vi "Configure Generator State.vi"(8 "error in (no error)":errorcluster, 9 "State (Off)":bool, 10 "Instance (1)":i32=1 format="%.0g", 11 "VISA resource name":refnum<visa-resource-name>) -> (0 "error out":errorcluster, 3 "VISA resource name out":refnum<visa-resource-name>)   [LabVIEW 2020, in "Rohde&Schwarz CMXP GPRF.lvlib"]
doc: "Turns the generator on or off.\n\nAttribute:\nRSCMXPGPRF_ATTR_GENERATOR_STATE\n\nRemote-control command:\nSOURce:GPRF:GEN<i>:STATe"
uses:
  <instrlib>/Rohde&Schwarz CMXP GPRF/Rohde&Schwarz CMXP GPRF.lvlib
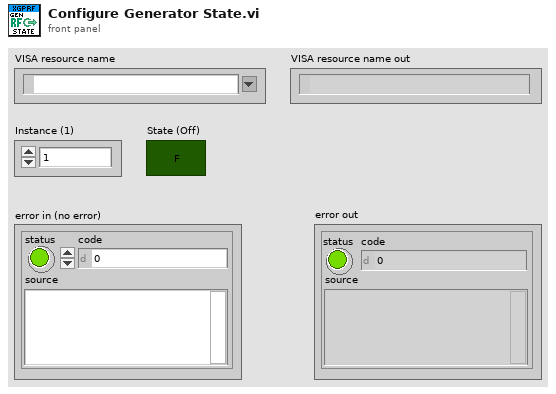
[diagram p1: front panel]
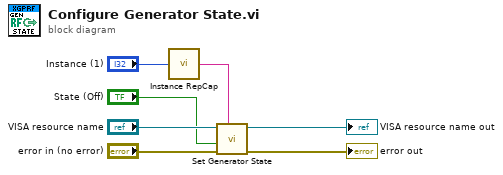
[diagram p0: block diagram]
diagram:
  n1 = call <instrlib>:"Instance RepCap.vi"("Instance in"="Instance (1)") -> ("Instance out"=w7:string)
  n2 = call "Set Generator State"("Repeated Capabilities"=w7, "error in (no error)"="error in (no error)", "Generator State (OFF)"="State (Off)", "instrument handle"="VISA resource name") -> ("error out"=→"error out":errorcluster, "instrument handle out"=→"VISA resource name out":refnum<visa-resource-name>)  [unwired: 6 in]
